vi "CalculateFFT.vi"(10 "Block Size":i32=-1, 11 "waveform":waveform(dbl)) -> (2 "FFT- Phase":cluster{dbl, dbl, dbl[]}(graph), 3 "FFT- Mag":cluster{dbl, dbl, dbl[]}(graph))   [LabVIEW 2022 SP3]
uses:
  <vilib>/Analysis/4window.llb/windowTd.ctl
  <vilib>/Analysis/2dsp.llb/Real FFT.vi
  <vilib>/measure/maspectr.llb/FFT Spectrum (Mag-Phase) for 1 Chan.vi
  <vilib>/Analysis/NI_AALPro.lvlib
  <vilib>/measure/NI_MAPro.lvlib
panel:
  out "FFT- Phase 2":cluster{"f0":dbl, "df":dbl, "phase":dbl[]}[](graph)
  out "FFT- Mag 2":cluster{"f0":dbl, "df":dbl, "magnitude":dbl[]}[](graph)
  # "Intput"
  # "Output"
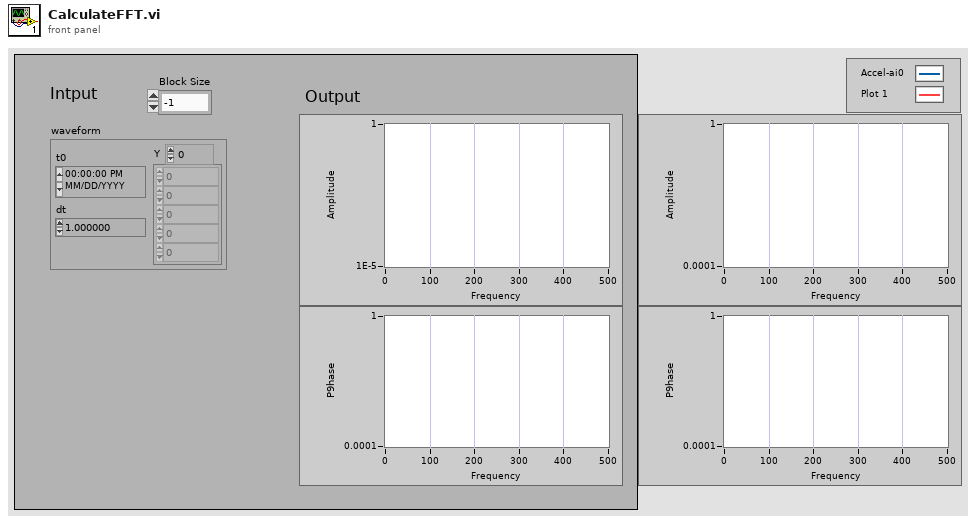
[diagram p1: front panel]
types:
  T1 = cluster{"averaging mode":enum16{"No averaging", "Vector averaging", "RMS averaging", "Peak hold"}, "weighting mode":enum16{"Linear", "Exponential"}, "number of averages":u32}
  T2 = cluster{"dB On (F)":bool, "unwrap phase (F)":bool, "convert to degree (F)":bool}
  T3 = typedef "NI_AALPro.lvlib/windowTd.ctl" = u32
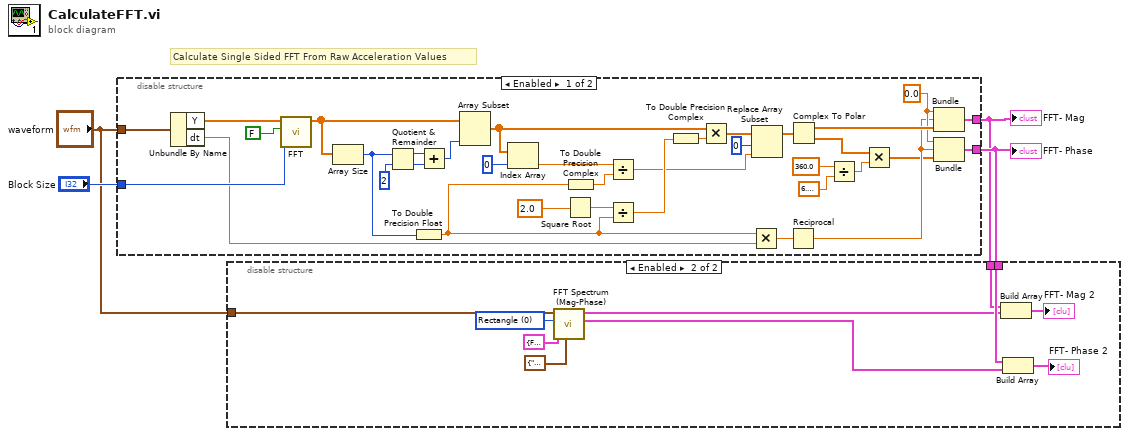
[diagram p0: block diagram]
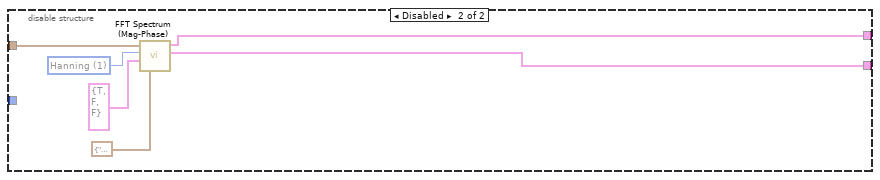
[diagram p3: hidden frame]
diagram:
  # "Calculate Single Sided FFT From Raw Acceleration Values"
  n1 = disable-structure shown="Enabled" {
    disable-tunnel: "Block Size" -> [w39 _]
    disable-tunnel: "waveform" -> [w5 w45]
    disable-tunnel: [w38 w40] -> w2
    disable-tunnel: [w37 w41] -> w1
    frame Enabled {
      w16 = 0.0
      n2 = Unbundle By Name(w5) -> ("Y"=w19:dbl[], "dt"=w12:dbl)
      n3 = call-poly <vilib>:"FFT.vi"("FFT size"=w39, "shift?"=FALSE, "X"=w19) -> ("FFT {X}"=w21:cdb[])  [unwired: 7 in, 1 out]
      n4 = Array Size(array=w21) -> (size(s)=w27:i32)
      n5 = Quotient & Remainder(x=w27, y=2) -> (x-y*floor(x/y)=w33:i32, floor(x/y)=w32:i32)
      n6 = To Double Precision Float(number=w27) -> (double precision float=w11:dbl)
      n7 = Add(x=w33, y=w32) -> (x+y=w31:i32)
      n8 = Array Subset(array=w21, length=w31) -> (w26:cdb[])  [unwired: 1 in]
      n9 = Index Array(array=w26, index=0) -> (element=w23:cdb)
      n10 = Square Root(x=2.0) -> (sqrt(x)=w14:dbl)
      n11 = To Double Precision Complex(1:w11) -> (0:w13:cdb)
      n12 = Divide(x=w23, y=w13) -> (x/y=w22:cdb)
      n13 = Divide(x=w14, y=w11) -> (x/y=w28:dbl)
      n14 = To Double Precision Complex(1:w28) -> (0:w30:cdb)
      n15 = Multiply(x=w26, y=w30) -> (x*y=w29:cdb[])
      n16 = Multiply(x=w11, y=w12) -> (x*y=w18:dbl)
      n17 = Replace Array Subset(array=w29, new element=w22, index=0 ("Index")) -> (w20:cdb[])
      n18 = Reciprocal(x=w18) -> (1/x=w15:dbl)
      n19 = Complex To Polar(r * e^(i*theta)=w20) -> (r=w17:dbl[], theta=w7:dbl[])
      n20 = Divide(x=360.0, y=6.283185307179586) -> (x/y=w9:dbl)
      n21 = Multiply(x=w7, y=w9) -> (x*y=w6:dbl[])
      n22 = Bundle(w16, w15, w17) -> (w37:cluster{dbl, dbl, dbl[]})  [unwired: 1 in]
      n23 = Bundle(w16, w15, w6) -> (w38:cluster{dbl, dbl, dbl[]})  [unwired: 1 in]
    }
    frame Disabled {
      w44 = T3 1 items=["Rectangle"=0, "Hanning"=1, "Hamming"=2, "Blackman-Harris"=3, "Exact Blackman"=4, "Blackman"=5, "Flat Top"=6, "4 Term B-Harris "=7, "7 Term B-Harris"=8, "Low Sidelobe"=9, "Blackman Nuttall"=11, "Triangle"=30, "Bartlett-Hanning"=31, "Bohman"=32, "Parzen"=33, "Welch"=34, "Kaiser"=60, "Dolph-Chebyshev"=61, "Gaussian"=62] ("window")
      n24 = call-poly <vilib>:"FFT Spectrum (Mag-Phase).vi"("averaging parameters"=T1 {"averaging mode"=enum."No averaging", "weighting mode"=enum."Linear", "number of averages"=2}, "view"=T2 {"dB On (F)"=TRUE, "unwrap phase (F)"=FALSE, "convert to degree (F)"=FALSE}, "window"=w44, "time signal"=w45) -> ("phase"=w40:cluster{"f0":dbl, "df":dbl, "phase":dbl[]}, "magnitude"=w41:cluster{"f0":dbl, "df":dbl, "magnitude":dbl[]})  [unwired: 3 in, 3 out]
    }
  }
  "FFT- Mag" <- w1
  "FFT- Phase" <- w2
  n25 = disable-structure shown="Enabled" {
    disable-tunnel: "waveform" -> [_ w55]
    disable-tunnel: w2 -> [_ w49]
    disable-tunnel: w1 -> [_ w47]
    frame Disabled {
    }
    frame Enabled {
      w54 = T3 0 items=["Rectangle"=0, "Hanning"=1, "Hamming"=2, "Blackman-Harris"=3, "Exact Blackman"=4, "Blackman"=5, "Flat Top"=6, "4 Term B-Harris "=7, "7 Term B-Harris"=8, "Low Sidelobe"=9, "Blackman Nuttall"=11, "Triangle"=30, "Bartlett-Hanning"=31, "Bohman"=32, "Parzen"=33, "Welch"=34, "Kaiser"=60, "Dolph-Chebyshev"=61, "Gaussian"=62] ("window")
      n26 = call-poly <vilib>:"FFT Spectrum (Mag-Phase).vi"("averaging parameters"=T1 {"averaging mode"=enum."No averaging", "weighting mode"=enum."Linear", "number of averages"=2}, "view"=T2 {"dB On (F)"=FALSE, "unwrap phase (F)"=FALSE, "convert to degree (F)"=FALSE}, "window"=w54, "time signal"=w55) -> ("phase"=w48:cluster{"f0":dbl, "df":dbl, "phase":dbl[]}, "magnitude"=w46:cluster{"f0":dbl, "df":dbl, "magnitude":dbl[]})  [unwired: 3 in, 3 out]
      n27 = Build Array(w47, w46) -> (→"FFT- Mag 2":cluster{"f0":dbl, "df":dbl, "magnitude":dbl[]}[])
      n28 = Build Array(w49, w48) -> (→"FFT- Phase 2":cluster{"f0":dbl, "df":dbl, "phase":dbl[]}[])
    }
  }
